vi "ac_measurement.vi"(8 "error in (no error)":errorcluster, 11 "UI in":T1) -> (0 "error out":errorcluster, 2 "element":dbl, 3 "output cluster":T1)   [LabVIEW 2017]
uses:
  ui.ctl
  ui_buttons.ctl
  <instrlib>/PICOTEST M352XA/Public/Controls/Function.ctl
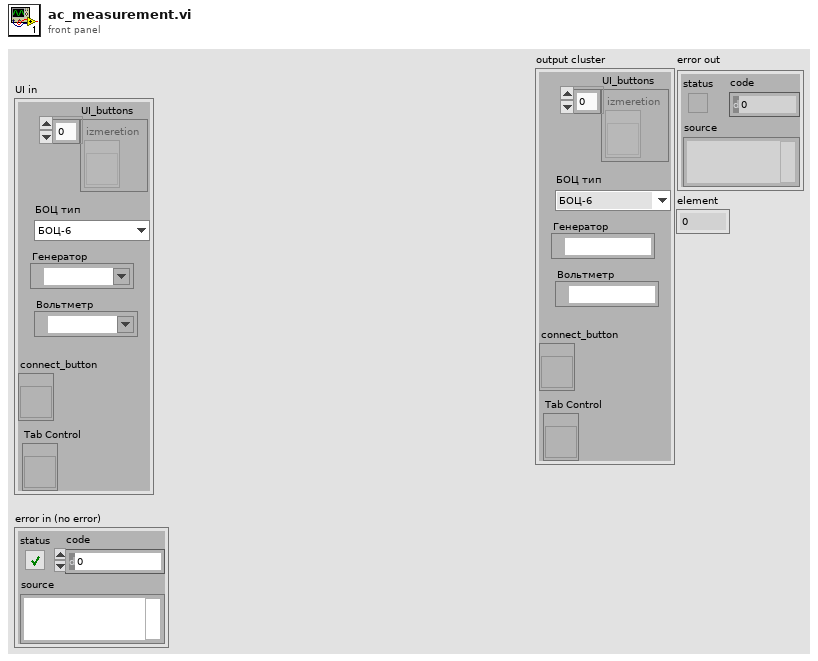
[diagram p1: front panel]
types:
  T1 = typedef "ui.ctl" = cluster{"UI_buttons":T2, "Tab Control":refnum<vi>, "connect_button":refnum<vi>, "boc_type":enum16{"БОЦ-6", "БОЦ-12"}, "generator":refnum<visa-resource-name>, "voltmetr":refnum<visa-resource-name>}
  T2 = typedef "ui_buttons.ctl" = refnum<vi>[]
  T3 = typedef "Function.ctl" = enum16{"VOLTage:DC", "VOLTage:DC:RATio", "VOLTage:AC", "CURRent:DC", "CURRent:AC", "RESistance", "FRESistance", "FREQuency", "PERiod", "FREQuency:CURRent", "PERiod:CURRent", "CAPacitance", "CONTinuity", "DIODe", "TCOuple", "TEMPerature"}
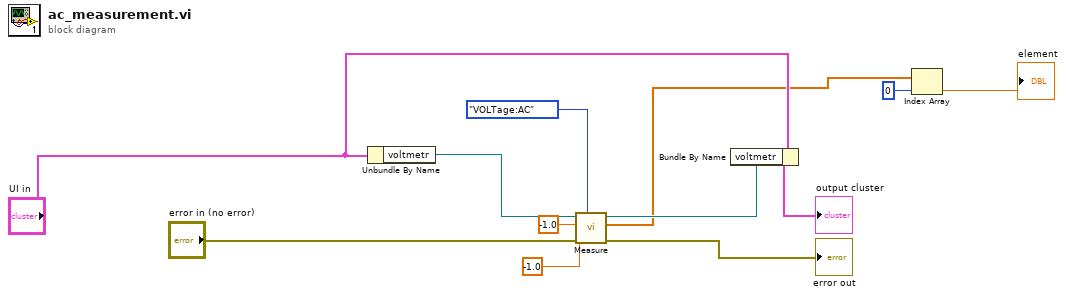
[diagram p0: block diagram]
diagram:
  n1 = Unbundle By Name("UI in") -> ("voltmetr"=w8:refnum<visa-resource-name>)
  n2 = call <instrlib>:"Measure.vi"("Function"=Function."VOLTage:AC", "error in (no error)"="error in (no error)", "Resolution"=-1.0, "Range"=-1.0, "VISA resource name"=w8) -> ("error out"=→"error out":errorcluster, "Measurements"=w3:dbl[], "VISA resource name out"=w11:refnum<visa-resource-name>)  [unwired: 4 in]
  n3 = Bundle By Name(cluster="UI in", "voltmetr"=w11) -> (→"output cluster":T1)
  n4 = Index Array(array=w3, index=0) -> (element=→"element":dbl)
